vi "Write.vi"(8 "error in (no error)":errorcluster, 10 "state data":T1, 11 "State in":refnum<class "State.lvclass">) -> (0 "error out":errorcluster, 3 "State out":refnum<class "State.lvclass">)   [LabVIEW 2019, in "DSF Core.lvlib" / "State.lvclass"]
uses:
  State.lvclass
  State Data.ctl
  State.lvclass/State.ctl
  <vilib>/NI/Memory Manager/Classes/Pointer/Pointer.lvclass/Pointer.ctl
  <vilib>/NI/Memory Manager/Classes/Pointer/Pointer.lvclass
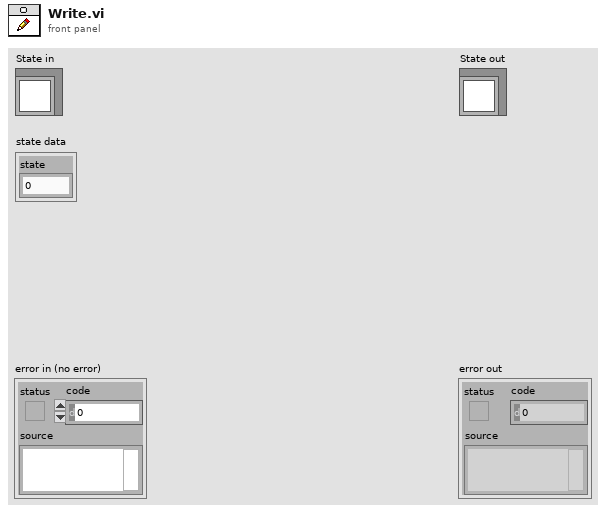
[diagram p1: front panel]
types:
  T1 = typedef "DSF Core.lvlib/State.lvclass/State Data.ctl" = cluster{"state":u8}
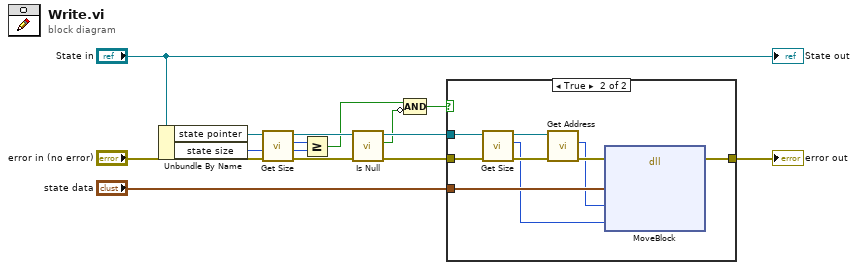
[diagram p0: block diagram]
diagram:
  n1 = Unbundle By Name("State in") -> ("state pointer"=w10:refnum<class "Pointer.lvclass">, "state size"=w9:u64)
  n2 = call <vilib>:"Get Size.vi"("Pointer in"=w10) -> ("size"=w7:u64, "Pointer out"=w8:refnum<class "Pointer.lvclass">)  [unwired: 9 in]
  n3 = Greater Or Equal?(x=w7, y=w9) -> (x >= y?=w6:bool)
  n4 = call <vilib>:"Is Null.vi"("error in (no error)"="error in (no error)", "Pointer in"=w8) -> ("error out"=w3:errorcluster, "null?"=w2:bool, "Pointer out"=w4:refnum<class "Pointer.lvclass">)  [unwired: 7 in]
  n5 = Compound Arithmetic op=AND(w6, invert w2) -> (w5:bool)
  n6 = case shown="True" w5 {
    tunnel: w4 -> [_ w19]
    tunnel: w3 -> [w14 w20]
    tunnel: [w14 w17] -> w13
    tunnel: "state data" -> [_ w21]
    frame False {
    }
    frame True {
      n7 = call <vilib>:"Get Size.vi"("Pointer in"=w19) -> ("size"=w16:u64, "Pointer out"=w18:refnum<class "Pointer.lvclass">)  [unwired: 9 in]
      n8 = call <vilib>:"Get Address.vi"("Pointer in"=w18) -> ("address"=w15:u64)  [unwired: 9 in, 1 out]
      n9 = dll-call lib="LabVIEW" fn="MoveBlock"(error in=w20, "src"=w21, "dst"=w15, "size"=w16) -> (error out=w17:errorcluster)  [unwired: 6 in, 1 out]
    }
  }
  "error out" <- w13
  "State out" <- "State in"
